vi "Read JWT from File.vi"(8 "error in (no error)":errorcluster, 11 "JWT Path In":path) -> (0 "error out":errorcluster, 2 "JWT":string, 3 "JWT Path":path)   [LabVIEW 2018, in "JWT.lvlib"]
uses:
  JWT.lvlib
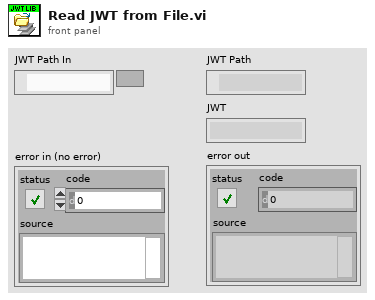
[diagram p1: front panel]
types:
  T1 = enum16{"open", "replace", "create", "open or create", "replace or create", "replace or create with confirmation"}
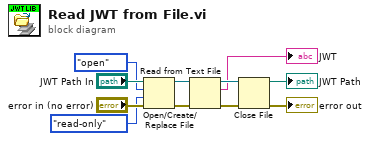
[diagram p0: block diagram]
diagram:
  n1 = Open/Create/Replace File(file path (use dialog)="JWT Path In", error in="error in (no error)", operation (0:open)=T1."open", access (0:read/write)=enum16{"read/write", "read-only", "write-only"}."read-only") -> (refnum out=w7:refnum<file>, error out=w6:errorcluster)  [unwired: 2 in, 1 out]
  n2 = Read from Text File(file (use dialog)=w7, error in=w6) -> (refnum out=w5:refnum<file>, text=→"JWT":string, error out=w4:errorcluster)  [unwired: 2 in, 1 out]
  n3 = Close File(refnum=w5, error in=w4) -> (path=→"JWT Path":path, error out=→"error out":errorcluster)
